vi "UltraForward.vi"(9 "RobotDriveDevRef":T3={"DevStatus"={"status"=FALSE, "code"=0, "source"=""}, "Motors[]"=[], "Square Inputs"=FALSE, "Max Output"=1.0, "Isochronous"=FALSE}, 10 "CounterDevRef in":T1, 11 "Target":dbl format="%#_13g") -> (1 "RobotDriveDevRef 2":T3={"DevStatus"={"status"=FALSE, "code"=0, "source"=""}, "Motors[]"=[], "Square Inputs"=FALSE, "Max Output"=1.0, "Isochronous"=FALSE})   [LabVIEW 2013]
uses:
  <vilib>/Rock Robotics/WPI/RobotDrive/WPI_RobotDriveDevRef.ctl
  <vilib>/Rock Robotics/WPI/MotorControl/WPI_MotorControlDeviceRef.ctl
  <vilib>/Rock Robotics/SystemInterfaces/Typedef/FPGA_TypedefDigitalModule.ctl
  <vilib>/Rock Robotics/SystemInterfaces/DIO/FPGA_DIOPWMChannel.ctl
  <vilib>/Rock Robotics/WPI/PWM/WPI_PWMDeadband.ctl
  <vilib>/Rock Robotics/WPI/CAN/Jaguar/SubVIs/WPI_CANJaguar_ControlMode.ctl
  <vilib>/Rock Robotics/WPI/PWM/WPI_PWMTransform_ConPane.ctl
  <vilib>/Rock Robotics/WPI/Counter/WPI_CounterDevRef.ctl
  <vilib>/Rock Robotics/SystemInterfaces/Counter/FPGA_CounterCtrSystemIndex.ctl
  <vilib>/addons/control/pid/pid.llb/PID (DBL).vi
  <vilib>/addons/control/pid/NI_PID_pid.lvlib
panel:
  out "CounterDevRef in 2":T1
  in  "Start?":bool=TRUE
  out "Array":dbl[](array[numeric])
  in  "output range 2":cluster{"output high":dbl, "output low":dbl}={"output high"=0.55, "output low"=-0.55}
  in  "PID gains 2":T11={"proportional gain (Kc)"=0.15, "integral time (Ti, min)"=0.0, "derivative time (Td, min)"=0.0}
  # "Stop?"
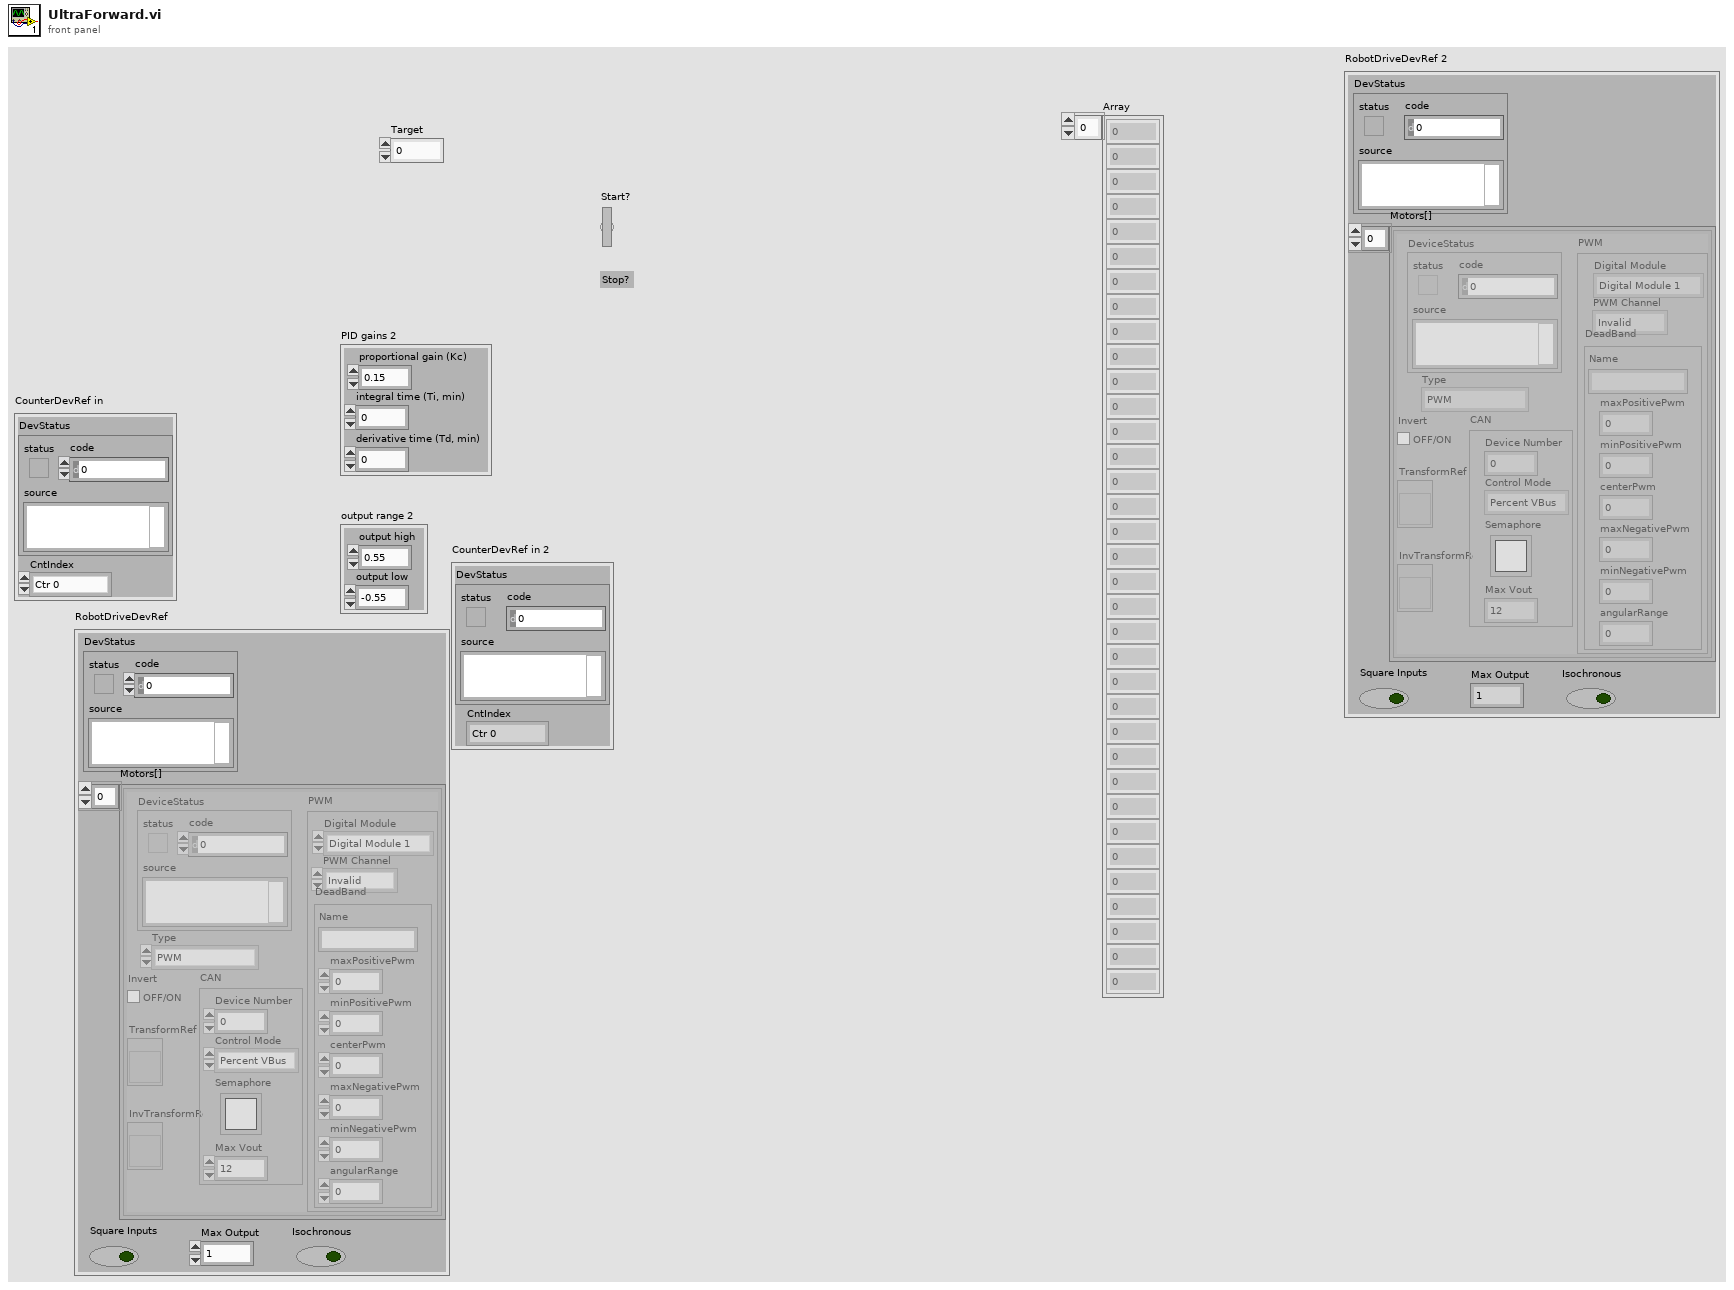
[diagram p1: front panel]
types:
  T1 = typedef "WPI_CounterDevRef.ctl" = cluster{"DevStatus":errorcluster, "CntIndex":T2}
  T2 = typedef "FPGA_CounterCtrSystemIndex.ctl" = enum8{"Ctr 0", "Ctr 1", "Ctr 2", "Ctr 3", "Ctr 4", "Ctr 5", "Ctr 6", "Ctr 7", "Invalid"}
  T3 = typedef "WPI_RobotDriveDevRef.ctl" = cluster{"DevStatus":errorcluster, "Motors[]":T4[], "Square Inputs":bool, "Max Output":dbl, "Isochronous":bool}
  T4 = typedef "WPI_MotorControlDeviceRef.ctl" = cluster{"DeviceStatus":errorcluster, "Type":enum16{"PWM", "CAN"}, "PWM":cluster{"Digital Module":T5, "PWM Channel":T6, "DeadBand":T7}, "CAN":cluster{"Device Number":u8, "Control Mode":T8, "Semaphore":T9, "Max Vout":dbl}, "Invert":bool, "TransformRef":T10, "InvTransformRef":T10}
  T5 = typedef "FPGA_TypedefDigitalModule.ctl" = enum16{"Digital Module 1", "Digital Module 2"}
  T6 = typedef "FPGA_DIOPWMChannel.ctl" = enum8{"PWM 1", "PWM 2", "PWM 3", "PWM 4", "PWM 5", "PWM 6", "PWM 7", "PWM 8", "PWM 9", "PWM 10", "Invalid"}
  T7 = typedef "WPI_PWMDeadband.ctl" = cluster{"Name":string, "maxPositivePwm":i32, "minPositivePwm":i32, "centerPwm":i32, "maxNegativePwm":i32, "minNegativePwm":i32, "angularRange":u16}
  T8 = typedef "WPI_CANJaguar_ControlMode.ctl" = enum8{"Percent VBus", "Current", "Speed", "Position", "Voltage"}
  T9 = typedef "Semaphore RefNum" = refnum<k1>
  T10 = typedef "WPI_PWMTransform_ConPane.ctl" = refnum<vi>
  T11 = cluster{"proportional gain (Kc)":dbl, "integral time (Ti, min)":dbl, "derivative time (Td, min)":dbl}
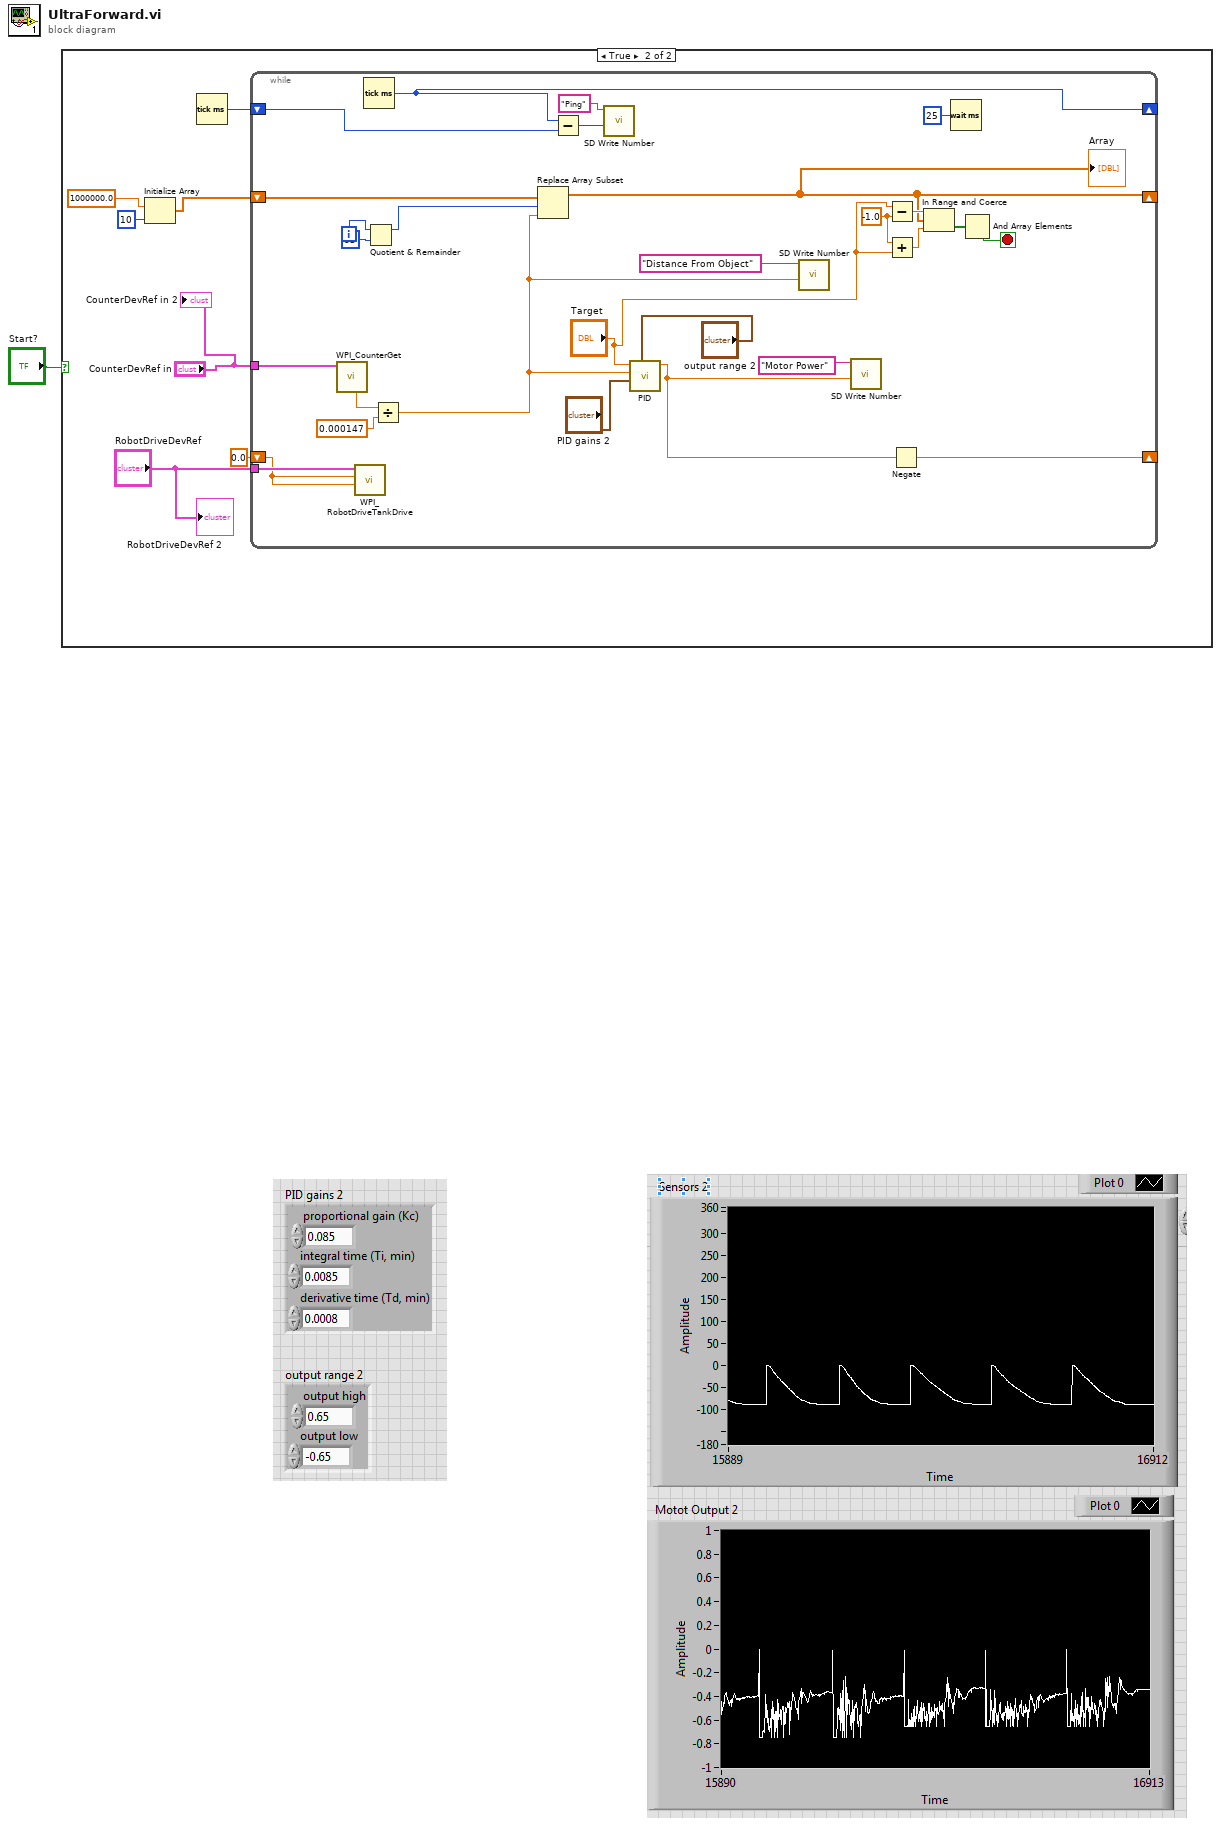
[diagram p0: block diagram]
diagram:
  n1 = case shown="True" "Start?" {
    frame False {
    }
    frame True {
      n2 = Initialize Array(1000000.0 ("element"), 10 ("dimension size")) -> (w4:dbl[])
      n3 = Tick Count (ms)() -> (millisecond timer value=w8:u32)
      n4 = while {
        shift-right: [w33] -> _
        shift-left: w8 -> [w34]
        shift-right: [w9] -> _
        shift-left: 0.0 ("output") -> [w14]
        tunnel: "RobotDriveDevRef" -> [w32]
        shift-right: [w18] -> _
        shift-left: w4 -> [w28]
        tunnel: "CounterDevRef in" -> [w11]
        i -> [w20]
        stop <- w26 stop-if-true
        w16 = -1.0 ("y")
        n5 = call <vilib>:"WPI_CounterGet.vi"("CounterDevRef in"=w11) -> ("Period (sec)"=w12:dbl)  [unwired: 5 in, 5 out]
        n6 = call <vilib>:"WPI_RobotDriveTankDrive.vi"("Right axis value"=w14, "Left axis value"=w14, "RobotDriveDevRef"=w32) -> ()  [unwired: 6 in, 3 out]
        n7 = Tick Count (ms)() -> (millisecond timer value=w33:u32)
        n8 = Quotient & Remainder(x=w20, y=35) -> (x-y*floor(x/y)=w29:i32)  [unwired: 1 out]
        n9 = Divide(x=w12, y=0.000147 ("Scaling factor (s/in)")) -> (x/y=w10:dbl)
        n10 = Replace Array Subset(array=w28, new element=w10, index=w29) -> (w18:dbl[])
        "Array" <- w18
        n11 = Subtract(x=w33, y=w34) -> (x-y=w24:u32)
        n12 = call <vilib>:"SD Write Number.vi"("Numeric"=w24, "Name"="Ping") -> ()  [unwired: 8 in, 2 out]
        n13 = call-poly <vilib>:"PID.vi"("output range"="output range 2", "PID gains"="PID gains 2", "process variable"=w10, "setpoint"="Target") -> ("output"=w22:dbl)  [unwired: 6 in, 1 out]
        n14 = call <vilib>:"SD Write Number.vi"("Numeric"=w10, "Name"="Distance From Object") -> ()  [unwired: 8 in, 2 out]
        n15 = call <vilib>:"SD Write Number.vi"("Numeric"=w22, "Name"="Motor Power") -> ()  [unwired: 8 in, 2 out]
        n16 = Subtract(x="Target", y=w16) -> (x-y=w27:dbl)
        n17 = Add(x=w16, y="Target") -> (x+y=w17:dbl)
        n18 = Negate(x=w22) -> (-x=w9:dbl)
        n19 = In Range and Coerce(upper limit=w27, x=w18, lower limit=w17) -> (In Range?=w19:bool[])  [unwired: 1 out]
        n20 = Wait (ms)(milliseconds to wait=u32 25) -> ()  [unwired: 1 out]
        n21 = And Array Elements(Boolean array=w19) -> (logical AND=w26:bool)
      }
      "RobotDriveDevRef 2" <- "RobotDriveDevRef"
      "CounterDevRef in 2" <- "CounterDevRef in"
    }
  }
